vi "Parse Condition Register.vi"(10 "Condition_Register":i16) -> (2 "Status_Flags":T1)   [LabVIEW 2019, in "3300.lvlib" / "3300.lvclass"]
uses:
  Library/3300.lvclass
  builds/Instruments/Electronic Load.lvlibp/Custom Controls/Status_Flags.ctl
  Custom Controls/Status_Register.ctl
  builds/Instruments/Electronic Load.lvlibp/Library/Electronic Load.lvclass
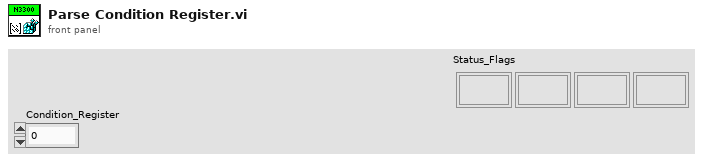
[diagram p1: front panel]
types:
  T1 = typedef "Electronic Load.lvlibp/Electronic Load.lvclass/Status_Flags.ctl" = cluster{"Interlock":bool, "OVP":bool, "OCP":bool, "Output":bool}
  T2 = typedef "3300.lvlib/3300.lvclass/Status_Register.ctl" = cluster{"Voltage Fault":bool, "Overcurrent":bool, "Spare_02":bool, "Overpower":bool, "Overtemperature":bool, "Spare_05":bool, "Spare_06":bool, "Spare_07":bool, "ReverseVoltageSens":bool, "ExtendedPowerUnavailable":bool, "InputUnregulated":bool, "ReverseVoltageIn":bool, "Overvoltage":bool, "Protection_Shutdown":bool, "Spare_14":bool, "Spare_15":bool}
  T3 = cluster{"Boolean array[0]":bool, "Boolean array[1]":bool, "Boolean array[2]":bool, "Boolean array[3]":bool, "Boolean array[4]":bool, "Boolean array[5]":bool, "Boolean array[6]":bool, "Boolean array[7]":bool, "Boolean array[8]":bool, "Boolean array[9]":bool, "Boolean array[10]":bool, "Boolean array[11]":bool}
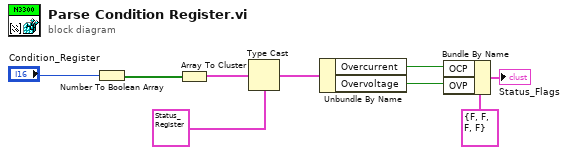
[diagram p0: block diagram]
diagram:
  n1 = Number To Boolean Array(number="Condition_Register") -> (Boolean array=w8:bool[])
  n2 = Array To Cluster(array=w8) -> (cluster=w7:T3)
  n3 = Type Cast(type=T2 {"Voltage Fault"=FALSE, "Overcurrent"=FALSE, "Spare_02"=FALSE, "Overpower"=FALSE, "Overtemperature"=FALSE, "Spare_05"=FALSE, "Spare_06"=FALSE, "Spare_07"=FALSE, "ReverseVoltageSens"=FALSE, "ExtendedPowerUnavailable"=FALSE, "InputUnregulated"=FALSE, "ReverseVoltageIn"=FALSE, "Overvoltage"=FALSE, "Protection_Shutdown"=FALSE, "Spare_14"=FALSE, "Spare_15"=FALSE} ("Status_Register"), x=w7) -> (*(type *) &x=w5:T2)
  n4 = Unbundle By Name(w5) -> ("Overcurrent"=w3:bool, "Overvoltage"=w2:bool)
  n5 = Bundle By Name(cluster=T1 {"Interlock"=FALSE, "OVP"=FALSE, "OCP"=FALSE, "Output"=FALSE} ("Status"), "OCP"=w3, "OVP"=w2) -> (→"Status_Flags":T1)
